vi "Actor Core.vi"(8 "error in":errorcluster, 11 "WebSocket Client in":refnum<class "WebSocket Client.lvclass">) -> (0 "error out":errorcluster, 3 "Actor out":refnum<class "Actor.lvclass">)   [LabVIEW 2017, in "WebSocket Client.lvlib" / "WebSocket Client.lvclass"]
doc: "(<B>Filename</B>: Actor Framework.lvlib:Actor.lvclass:Actor Core.vi)\n\nReceives messages to the actor, reacts to them, and initiates any error handling that may shut the actor down.\n\nDescendant classes may override this VI to append parallel tasks for the actor to complete while it handles messages. Overrides use the Call Parent Method node."
uses:
  WebSocket Client.lvclass
  <vilib>/ActorFramework/Actor/Actor.lvclass
  Framework/Actor wHelper/Actor wHelper.lvclass
panel:
  # "Headless WebSocket Client"
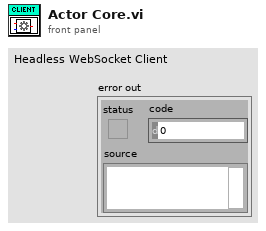
[diagram p1: front panel]
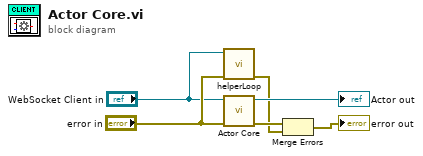
[diagram p0: block diagram]
diagram:
  n1 = call-dynamic "helperLoop.vi"("error in (no error)"="error in", "WebSocket Client in"="WebSocket Client in") -> ("error out"=w1:errorcluster)  [unwired: 8 in, 1 out]
  n2 = call-parent "Actor Core.vi"("error in"="error in", "Actor in"="WebSocket Client in") -> ("error out"=w6:errorcluster, "Actor out"=→"Actor out":refnum<class "Actor.lvclass">)  [unwired: 8 in]
  n3 = Merge Errors(w6, w1) -> (→"error out":errorcluster)
